vi "Configure.vi"(8 "error in (no error)":errorcluster, 11 "VacSys in":refnum<class "VacSys.lvclass">) -> (0 "error out":errorcluster, 3 "VacSys out":refnum<class "VacSys.lvclass">)   [LabVIEW 2018, in "VacSys.lvclass"]
uses:
  VacSys.lvclass
  VacSys.lvclass/VacSys.ctl
  <vilib>/Utility/config.llb/Read Key (String).vi
  GaugeFactory/GaugeFactory.lvclass
  <vilib>/Utility/config.llb/NI_LVConfig.lvlib
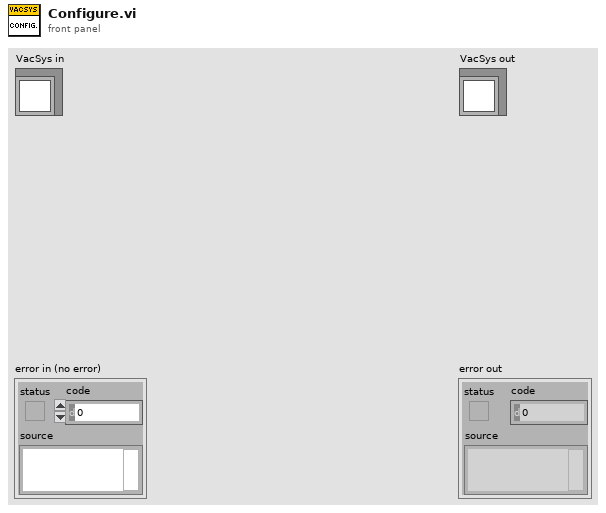
[diagram p1: front panel]
types:
  T1 = typedef "NI_LVConfig.lvlib/Config Data RefNum.ctl" = refnum<k1>
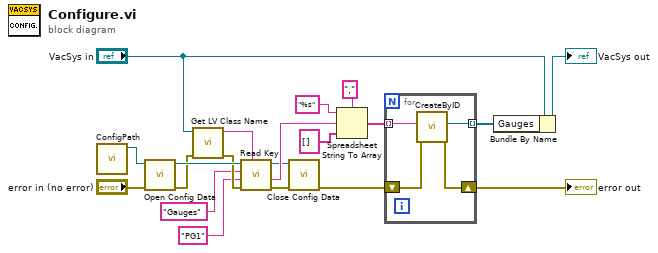
[diagram p0: block diagram]
diagram:
  n1 = call "ConfigPath.vi"() -> ("ConfigPath"=w17:path)  [unwired: 11 in]
  n2 = call <vilib>:"Open Config Data.vi"("error in (no error)"="error in (no error)", "configuration file path"=w17) -> ("error out"=w13:errorcluster, "refnum"=w16:T1)  [unwired: 7 in, 1 out]
  n3 = call <vilib>:"Get LV Class Name.vi"("error in (no error)"=w13, "object"="VacSys in") -> ("error out"=w9:errorcluster, "class name"=w14:string)  [unwired: 8 in]
  n4 = call-poly <vilib>:"Read Key.vi"("section"=w14, "error in (no error)"=w9, "default value"="PG1" ("key"), "key"="Gauges", "refnum"=w16) -> ("error out"=w11:errorcluster, "value"=w6:string, "refnum out"=w1:T1)  [unwired: 3 in, 1 out]
  n5 = call <vilib>:"Close Config Data.vi"("error in (no error)"=w11, "refnum"=w1) -> ("error out"=w10:errorcluster)  [unwired: 8 in, 1 out]
  n6 = Spreadsheet String To Array(delimiter (Tab)=",", format string="%s", spreadsheet string=w6, array type (2D Dbl)=string[] [] ("GaugeType")) -> (array=w5:string[])
  n7 = for {
    tunnel: [w24] -> w19 mode=indexing
    shift-right: [w21] -> w18
    shift-left: w10 -> [w22]
    tunnel: w5 -> [w23] mode=indexing
    n8 = call "CreateByID.vi"("error in (no error)"=w22, "GaugeID"=w23) -> ("error out"=w21:errorcluster, "IGauge"=w24:refnum<class "IGauge.lvclass">)  [unwired: 7 in, 1 out]
  }
  "error out" <- w18
  n9 = Bundle By Name(cluster="VacSys in", "Gauges"=w19) -> (→"VacSys out":refnum<class "VacSys.lvclass">)
